vi "_EnumEditor_GetVIref.vi"(8 "error in (no error)":errorcluster, 11 "_EnumEditor in":refnum<class "_EnumEditor.lvclass">) -> (0 "error out":errorcluster, 2 "Vi ref":refnum<vi>, 3 "_EnumEditor out":refnum<class "_EnumEditor.lvclass">)   [LabVIEW 2014, in "_EnumEditor.lvclass"]
uses:
  _EnumEditor.lvclass
  _EnumEditor.lvclass/_EnumEditor.ctl
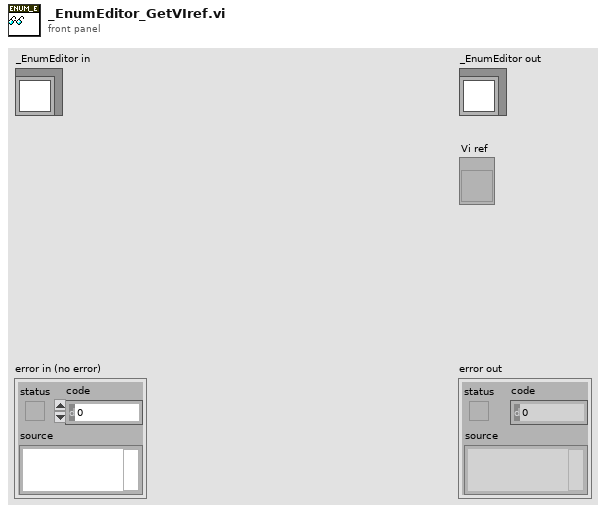
[diagram p1: front panel]
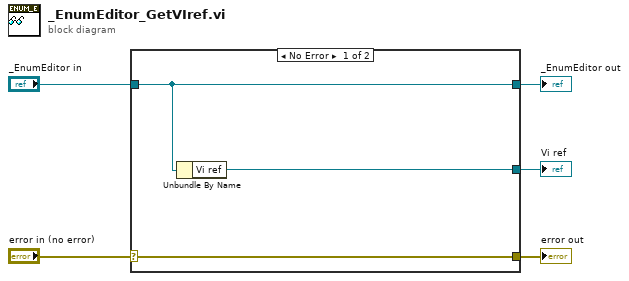
[diagram p0: block diagram]
diagram:
  n1 = case shown="No Error" "error in (no error)" {
    selector: "error in (no error)" -> [w8 w9]
    tunnel: [w8 w9] -> w4
    tunnel: [w7 w10] -> w2
    tunnel: "_EnumEditor in" -> [w7 w10]
    tunnel: [w6 _] -> w1
    frame No Error {
      n2 = Unbundle By Name(w7) -> ("Vi ref"=w6:refnum<vi>)
    }
    frame Error {
    }
  }
  "error out" <- w4
  "_EnumEditor out" <- w2
  "Vi ref" <- w1
